vi "Log Event.vi"(6 "Event Time":timestamp, 7 "Event Level":T1, 8 "error in (no error)":errorcluster, 10 "Data To Log":string, 11 "SourceID":string) -> (0 "error out":errorcluster)   [LabVIEW 2018, in "MVA Framework.lvlib" / "Singleton Event Log.lvlib"]
uses:
  Singleton Event Log.lvlib
  LoggerReference/LoggerReference.lvclass
  Types/Log Level.ctl
  Composed Log.lvlib
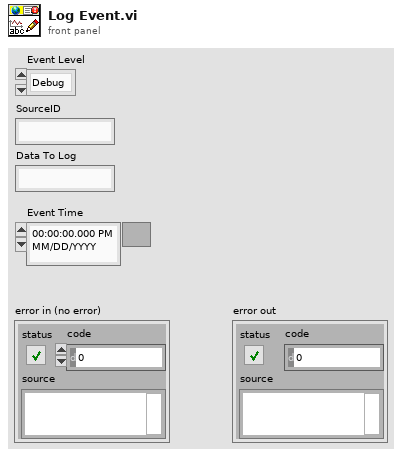
[diagram p1: front panel]
types:
  T1 = typedef "MVA Framework.lvlib/Composed Log.lvlib/Log Level.ctl" = enum16{"Debug", "Info", "Warning", "Error", "Critical"}
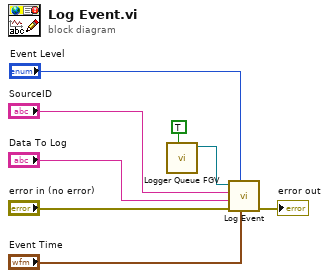
[diagram p0: block diagram]
diagram:
  n1 = call "Logger Queue FGV.vi"("Read?"=TRUE) -> ("LogReference Instance Out"=w2:refnum<class "LoggerReference.lvclass">)  [unwired: 10 in]
  n2 = call "Log Event.vi"("Event Time"="Event Time", "Event Level"="Event Level", "error in (no error)"="error in (no error)", "Data To Log"="Data To Log", "SourceID"="SourceID", "Log Instance"=w2) -> ("error out"=→"error out":errorcluster)  [unwired: 4 in, 1 out]
